vi "rss.vi"(1 "Type B":dbl, 2 "Type A":dbl[](array[numeric])) -> (0 "U_c":dbl[](array[numeric]))   [LabVIEW 2021, in "CALIBRATION.lvlib"]
uses:
  CALIBRATION.lvlib
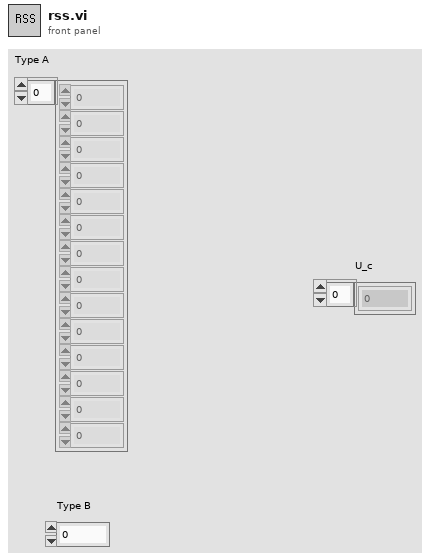
[diagram p1: front panel]
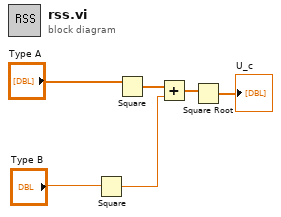
[diagram p0: block diagram]
diagram:
  n1 = Square(x="Type B") -> (x^2=w1:dbl)
  n2 = Square(x="Type A") -> (x^2=w3:dbl[])
  n3 = Add(x=w3, y=w1) -> (x+y=w5:dbl[])
  n4 = Square Root(x=w5) -> (sqrt(x)=→"U_c":dbl[])
